vi "FTW-Endpoint-CreateSender.vi"(0 "FTW Endpoint":refnum<class "FTW-Endpoint-TCP.lvclass">, 5 "Endpoint Address":string, 9 "Buffer Depth (1)":i32=1, 11 "error in":errorcluster) -> (4 "FTW Endpoint out":refnum<class "FTW-Endpoint-TCP.lvclass">, 15 "error out":errorcluster)   [LabVIEW 2015, in "FTW-Endpoint-TCP.lvclass"]
uses:
  FTW-Endpoint-TCP.lvclass
panel:
  # "Inputs"
  # "Outputs"
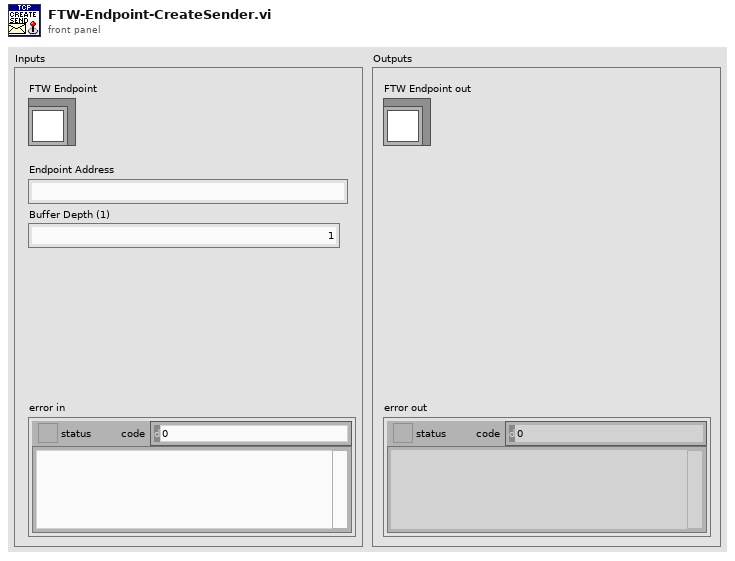
[diagram p1: front panel]
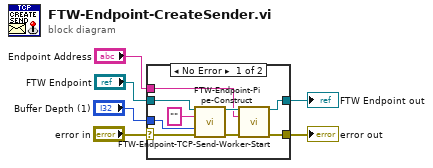
[diagram p0: block diagram]
diagram:
  n1 = case shown="No Error" "error in" {
    selector: "error in" -> [w13 w16]
    tunnel: "FTW Endpoint" -> [w12 w17]
    tunnel: [w14 w17] -> w4
    tunnel: [w15 w16] -> w3
    tunnel: "Endpoint Address" -> [w9 _]
    tunnel: "Buffer Depth (1)" -> [w7 _]
    frame No Error {
      n2 = call-dynamic "FTW-Endpoint-Pipe-Construct.vi"("FTW Endpoint"=w12, "Address"="", "Size (-1)"=w7, "error in"=w13) -> ("FTW Endpoint out"=w10:refnum<class "FTW-Endpoint-TCP.lvclass">, "error out"=w11:errorcluster)  [unwired: 9 in, 1 out]
      n3 = call-dynamic "FTW-Endpoint-TCP-Send-Worker-Start.vi"("FTW-Endpoint-TCP In"=w10, "Endpoint Address"=w9, "error in"=w11) -> ("FTW-Endpoint-TCP Out"=w14:refnum<class "FTW-Endpoint-TCP.lvclass">, "error out"=w15:errorcluster)  [unwired: 11 in]
    }
    frame Error {
    }
  }
  "error out" <- w3
  "FTW Endpoint out" <- w4
